vi "parse_PolynomialSegment.vi"   [LabVIEW 2018]
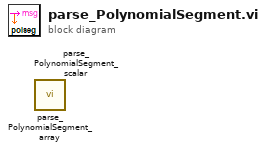
[diagram p0: block diagram]
diagram:
  n1 = call <userlib>:"parse_PolynomialSegment_array.vi"() -> ()  [unwired: 5 in, 3 out]
  n2 = call <userlib>:"parse_PolynomialSegment_scalar.vi"() -> ()  [unwired: 5 in, 3 out]
